vi "DiffDriveTrainSim_GetPose.vi"(11 "DiffDriveTrainSim":T4 {"m_Motor"."Jr_KgM2" format="%13.5p"; "m_Motor"."L_H" format="%13.5p"; "m_Motor"."Kt_NMPerAmp" format="%13.5p"; "m_Motor"."KvINV_RadPerSecPerVolt" format="%13.5p"; "m_Motor"."R_Ohms" format="%13.5p"; "m_Motor"."FreeSpeed_RadPerSec" format="%13.5p"; "m_Motor"."FreeCurrent_Amps" format="%13.5p"; "m_Motor"."StallCurrent_Amps" format="%13.5p"; "m_Motor"."StallTorque_NM" format="%13.5p"; "m_Motor"."nominalVoltage_Volts" format="%13.5p"}) -> (3 "Pose":T1={"TRANSLATION"={"X"=0.0, "Y"=0.0}, "ROTATION"={"VALUE"=0.0, "COS"=1.0, "SIN"=0.0}} {"ROTATION"."SIN" format="%13.4f"; "ROTATION"."COS" format="%13.4f"; "ROTATION"."VALUE" format="%13.4f"; "TRANSLATION"."Y" format="%14.3f"; "TRANSLATION"."X" format="%14.3f"})   [LabVIEW 2019, in "Trajectory_Library.lvlib"]
doc: "Returns the current pose.\n \nInputs:\n - DiffDriveTraimSim -- Data cluster\n\nOutputs:\n - Pose -- The current pose."
uses:
  Trajectory_Library.lvlib
  Enum/DIFF_DRIVE_TRAIN_SIM_STATE_ENUM.ctl
  TypeDef/LINEAR_SYSTEM.ctl
  <vilib>/Analysis/Matrix/Datatypes/RealMatrix.ctl
  <vilib>/Analysis/Matrix/NI_Matrix.lvlib
  TypeDef/DCMOTOR.CTL
  TypeDef/DIFF_DRIVE_TRAIN_SIM.ctl
  TypeDef/TRANSLATION2D.ctl
  TypeDef/ROTATION2D.ctl
  TypeDef/POSE2D.ctl
panel:
  # "<States, 1>"
  # "<Outputs, 1>"
  # "<Inputs, 1>"
  # "<Outputs, 1>"
  # "<States,States>"
  # "<States,Inputs>"
  # "<Outputs,States>"
  # "<Outputs,Inputs>"
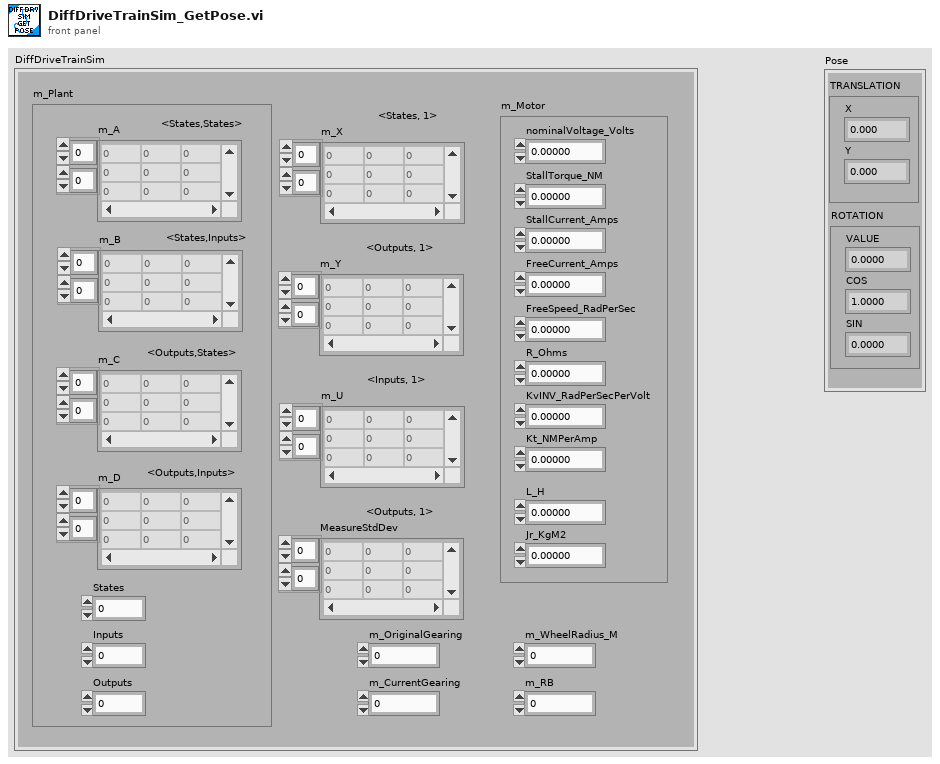
[diagram p1: front panel]
types:
  T1 = typedef "Trajectory_Library.lvlib/POSE2D.ctl" = cluster{"TRANSLATION":T2, "ROTATION":T3}
  T2 = typedef "Trajectory_Library.lvlib/TRANSLATION2D.ctl" = cluster{"X":dbl, "Y":dbl}
  T3 = typedef "Trajectory_Library.lvlib/ROTATION2D.ctl" = cluster{"VALUE":dbl, "COS":dbl, "SIN":dbl}
  T4 = typedef "Trajectory_Library.lvlib/DIFF_DRIVE_TRAIN_SIM.ctl" = cluster{"m_Plant":T5, "m_X":T6, "m_Y":T6, "m_U":T6, "MeasureStdDev":T6, "m_Motor":T7, "m_OriginalGearing":dbl, "m_CurrentGearing":dbl, "m_WheelRadius_M":dbl, "m_RB":dbl}
  T5 = typedef "Trajectory_Library.lvlib/LINEAR_SYSTEM.ctl" = cluster{"m_A":T6, "m_B":T6, "m_C":T6, "m_D":T6, "States":i32, "Inputs":i32, "Outputs":i32}
  T6 = typedef "NI_Matrix.lvlib/RealMatrix.ctl" = dbl[][]
  T7 = typedef "Trajectory_Library.lvlib/DCMOTOR.CTL" = cluster{"nominalVoltage_Volts":dbl, "StallTorque_NM":dbl, "StallCurrent_Amps":dbl, "FreeCurrent_Amps":dbl, "FreeSpeed_RadPerSec":dbl, "R_Ohms":dbl, "KvINV_RadPerSecPerVolt":dbl, "Kt_NMPerAmp":dbl, "L_H":dbl, "Jr_KgM2":dbl}
  T8 = typedef "Trajectory_Library.lvlib/DIFF_DRIVE_TRAIN_SIM_STATE_ENUM.ctl" = enum16{"X_POS", "Y_POS", "HEADING", "LEFT_VEL", "RIGHT_VEL", "LEFT_DIST", "RIGHT_DIST"}
  T9 = typedef "WPILib_Math.lvlib/POSE2D.ctl" = cluster{"TRANSLATION":T10, "ROTATION":T11}
  T10 = typedef "WPILib_Math.lvlib/TRANSLATION2D.ctl" = cluster{"X":dbl, "Y":dbl}
  T11 = typedef "WPILib_Math.lvlib/ROTATION2D.ctl" = cluster{"VALUE":dbl, "COS":dbl, "SIN":dbl}
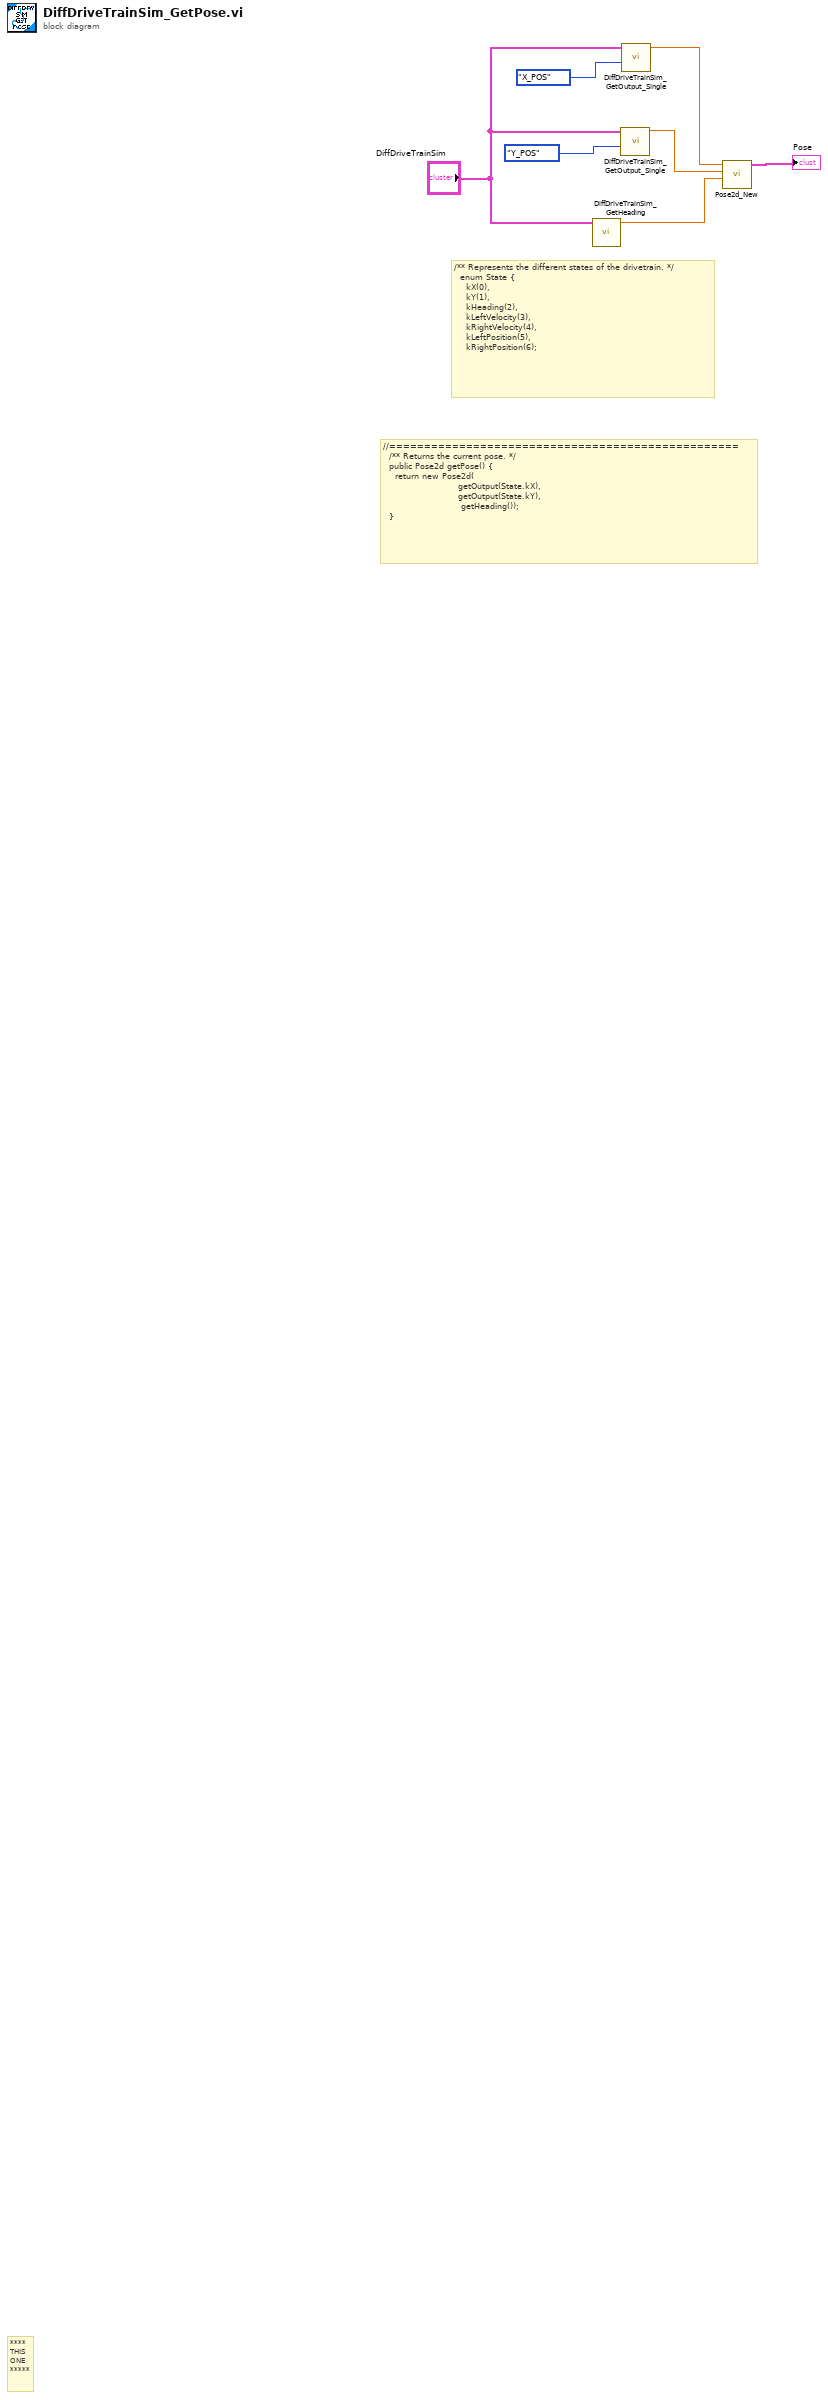
[diagram p0: block diagram]
diagram:
  # "/** Represents the different states of the drivetrain. */\n  enum State {\n    kX(0),\n    kY(1),\n    kHeading(2),\n    kLeftVelocity(3),\n    kRightVelocity(4),\n    kLeftPosition(5),\n    kRightPosition(6);"
  # "//==================================================\n  /** Returns the current pose. */\n  public Pose2d getPose() {\n    return new Pose2d(\n                         getOutput(State.kX), \n                         getOutput(State.kY), \n                          getHeading());\n  }"
  # "****\nTHIS\nONE\n*****"
  n1 = call "DiffDriveTrainSim_GetHeading.vi"("DiffDriveTrainSim"="DiffDriveTrainSim") -> ("Heading"=w7:dbl)  [unwired: 10 in]
  n2 = call "DiffDriveTrainSim_GetOutput_Single.vi"("Row"=DIFF_DRIVE_TRAIN_SIM_STATE_ENUM."Y_POS" ("DIFF_DRIVE_TRAIN_SIM_STATE"), "DiffDriveTrainSim"="DiffDriveTrainSim") -> ("Output"=w4:dbl)  [unwired: 9 in]
  n3 = call "DiffDriveTrainSim_GetOutput_Single.vi"("Row"=DIFF_DRIVE_TRAIN_SIM_STATE_ENUM."X_POS" ("DIFF_DRIVE_TRAIN_SIM_STATE"), "DiffDriveTrainSim"="DiffDriveTrainSim") -> ("Output"=w5:dbl)  [unwired: 9 in]
  n4 = call "Pose2d_New.vi"("Heading"=w7, "Y"=w4, "X"=w5) -> ("out POSe"=→"Pose":T9)  [unwired: 8 in]
